vi "gCode_Help.vi"(11 "Input String":string) -> (3 "stringOut":string="No help documentation at this time")   [LabVIEW 2015]
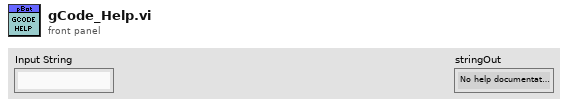
[diagram p1: front panel]
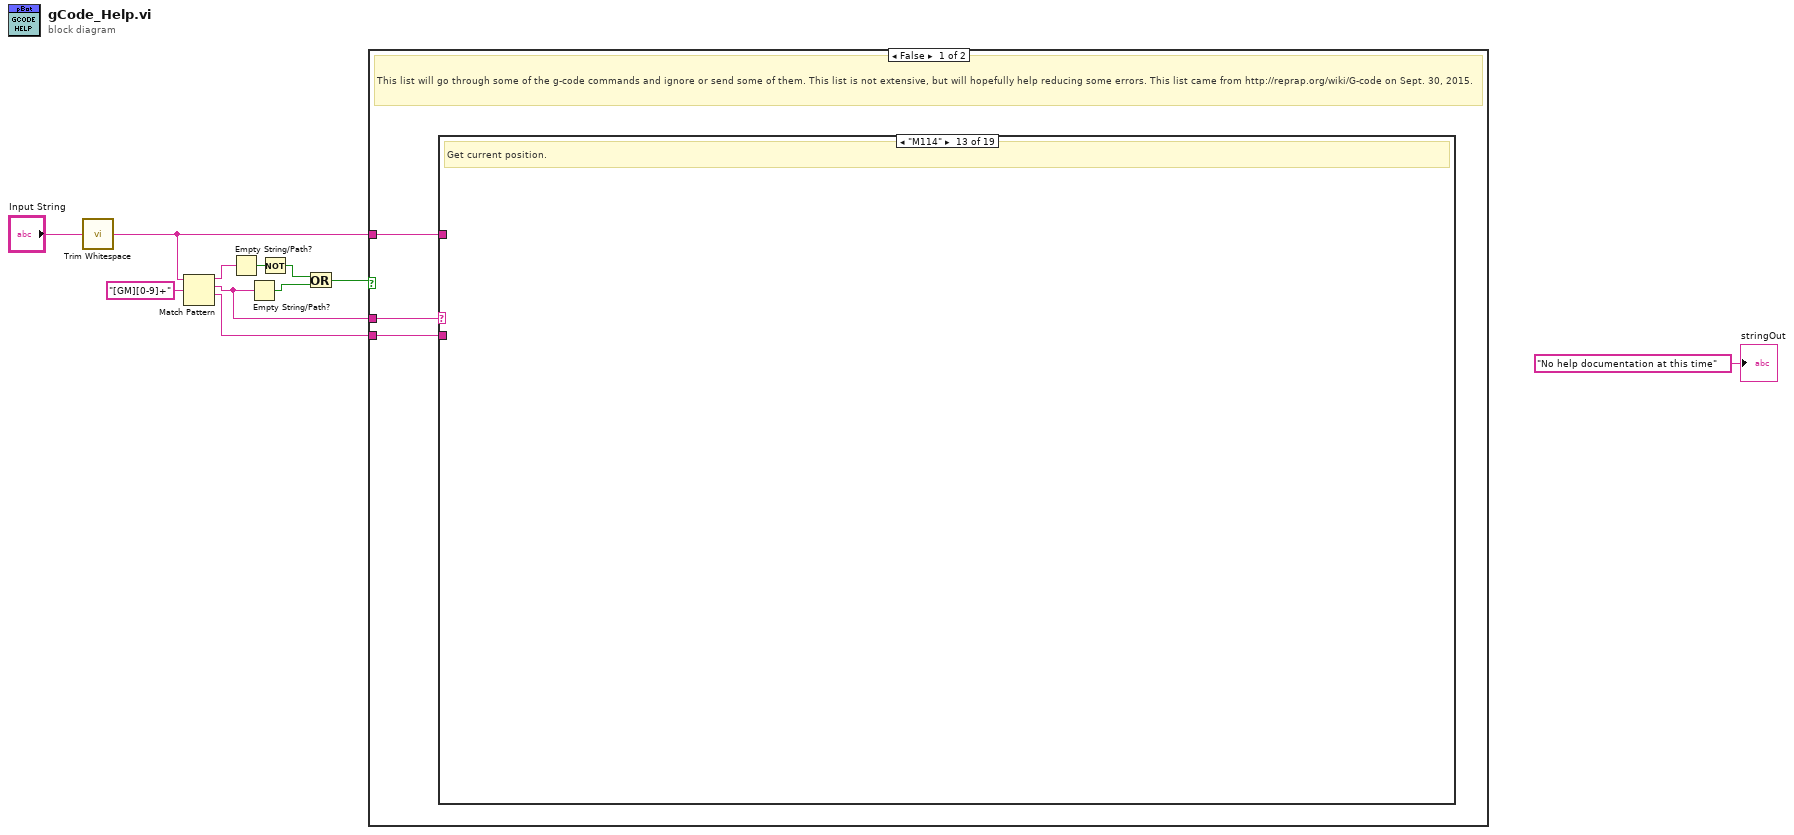
[diagram p0: block diagram]
diagram:
  n1 = call <vilib>:"Trim Whitespace.vi"("string"="Input String") -> ("trimmed string"=w2:string)  [unwired: 1 in]
  n2 = Match Pattern(string=w2, regular expression="[GM][0-9]+") -> (before substring=w9:string, match substring=w4:string, after substring=w3:string)  [unwired: 1 in, 1 out]
  n3 = Empty String/Path?(string/path=w9) -> (empty?=w8:bool)
  n4 = Empty String/Path?(string/path=w4) -> (empty?=w6:bool)
  n5 = Not(x=w8) -> (.not. x?=w7:bool)
  n6 = Or(x=w7, y=w6) -> (x .or. y?=w5:bool)
  n7 = case shown="False" w5 {
    tunnel: w4 -> [w14 _]
    tunnel: w3 -> [w13 _]
    tunnel: w2 -> [w12 _]
    frame False {
      # "This list will go through some of the g-code commands and ignore or send some of them. This list is not extensive, but will hopefully help reducing some errors. This list came from http://reprap.org/wiki/G-code on Sept. 30, 2015."
      n8 = case shown="\"M114\"" w14 {
        tunnel: w13 -> [_ _ _ _ _ _ _ _ _ _ _ _ _ _ _ _ _ _ _]
        tunnel: w12 -> [_ _ _ _ _ _ _ _ _ _ _ _ _ _ _ _ _ _ _]
        frame "G2", "G3" {
          # "These are controlled arc moves, and I will just skip all of these."
        }
        frame "G0", "G1" {
          # "Linear motion commands"
        }
        frame "G92" {
          # "Set position as"
        }
        frame "G90" {
          # "Set to absolute positioning"
        }
        frame "G91" {
          # "set to relative positioning"
        }
        frame "G29" {
          # "This command would measure the position of the bed in three positions and then fit those points to a plane. Using this plane, the firmware would correct for any unlevelness of the bed in real time. However, since the bed is not metal and the curent position of the probe is off the bed; this command is not allowed.\nAt some time, we should make a head mount to hold the z-sensor, and then put aluminum foil on the bed so that we can use this command. However, you would not want to do this everytime you turn the printer on, and I do not know if the values it measured are stored in the onboard memory between reboots and if it would automatically use the values. (In 3D printing this command is run betore every single 3d print and so it doesnt need to be stored.)"
        }
        frame "G28" {
          # "Home the axis -- note we need to home Y first then X and then Z. This is to reduce the posibitlity of the head colliding with any objects on the breadboard."
        }
        frame "M20", "M21", "M22", "M23", "M24", "M25", "M26", "M27", "M28", "M29", "M30", "M31", "M32", "M33", "M34", "M928" {
          # "These commands are all about SD cards and will be ignored."
        }
        frame "M104", "M108", "M109", "M207", "M221", "M82", "M83" {
          # "Commands about extruders that will be ignored.\nNote --- M83, M109 are about setting the temperature of the extruder. If a heater was installed (for instance for cell incumation) and the correct thermistor was used for measuring the temperature, then this command might be able to be used for setting that temperature."
        }
        frame "M105" {
          # "Get current extruder/bed temperature"
        }
        frame "M106", "M107" {
          # "Turn fan on or off. -- currently no fan installed"
        }
        frame "M112" {
          # "I don't know if I should do this or not, and I dont want to test it; so, for now it will be disabled"
          # "Emergancy stop. All moves immediately terminated, then all motors and heaters are turned off. To start again, need to press the master reset button on the printerBoard (says wikipedia -- never tried this command though."
        }
        frame "M114" {
          # "Get current position."
        }
        frame "M140", "M190" {
          # "Commands for setting temperature of heated bed -- no heated bed installed"
        }
        frame "M502" {
          # "Resets all tunable parameters to factory reset values."
        }
        frame "M501" {
          # "Read parameters from EEPROM"
        }
        frame "M500" {
          # "Save parameters to EEPROM"
        }
        frame "M600", "M605", "M665", "M668", "M999" {
          # "other commands to ignore"
        }
        frame Default {
          # "IF the command is not in this case structure, then ask the user to make sure they want to send the command to the printerboard"
        }
      }
    }
    frame True {
      # "Illegal gCode command. I require that a G or M command be the first thing in the string"
    }
  }
  "stringOut" <- "No help documentation at this time" ("regular expression")
